vi "Wash Display Console View.vi"(8 "error in (no error)":errorcluster, 11 "View Model":T2) -> (0 "error out":errorcluster)   [LabVIEW 2017]
doc: "Contains set of indicators for demonstrate current state of Car Wash process."
uses:
  View Model/Controls/View Model.ctl
  Configuration Database/Controls/Config Model.ctl
  Configuration Database/Controls/Config Commands.ctl
  Configuration Database/Controls/Congif Data.ctl
  View Model/Controls/Shared Model.ctl
  Error Handler/Controls/Error Model.ctl
  Error Handler/Controls/Error Data.ctl
  Error Handler/Controls/Error Type.ctl
  Car Wash Controller/Controls/Car Wash Model.ctl
  Car Wash Controller/Controls/Controller Overhead.ctl
  Car Wash Controller/Controls/Vehicle Location.ctl
  Car Wash Controller/Controls/Car Wash States.ctl
  Car Wash Controller/Controls/CarWash CMD.ctl
  Controls/Car Wash Indicators.ctl
panel:
  out "Time Remaining":dbl format="%07.2g"
  out "Vehicle Out of Position":bool
  out "Wash Entry":bool
  out "Car Wash Indicators":T1
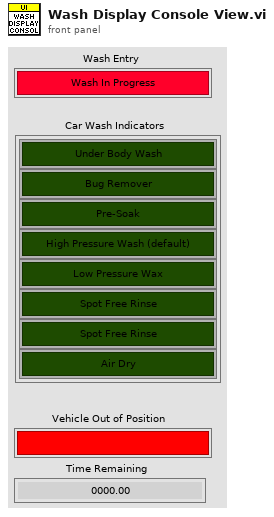
[diagram p1: front panel]
types:
  T1 = typedef "Car Wash Indicators.ctl" = cluster{"Under Body Wash":bool, "Bug Remover":bool, "Pre-Soak":bool, "High Pressure Wash":bool, "Low Pressure Wax":bool, "Spot Free Rinse":bool, "Tire Shine Foam":bool, "Air Dry":bool}
  T2 = typedef "View Model.ctl" = cluster{"Config Model":T3, "Shared Model":T4, "Error Model":T5, "Car Wash Model":T6}
  T3 = typedef "Config Model.ctl" = cluster{"Config CMD":refnum<user-event>, "Config Locked?":refnum<data-value>, "Config DVR":refnum<data-value>}
  T4 = typedef "Shared Model.ctl" = cluster{"Stop event":refnum<user-event>, "Stop DVR":refnum<data-value>}
  T5 = typedef "Error Model.ctl" = cluster{"Error event":refnum<user-event>}
  T6 = typedef "Car Wash Model.ctl" = cluster{"Out of Position Change":refnum<user-event>, "Wash Entry Change":refnum<user-event>, "Contr Overhead DVR":refnum<data-value>, "CarWash CMD":refnum<user-event>, "Location Change":refnum<user-event>, "Car Wash LEDs Change":refnum<user-event>}
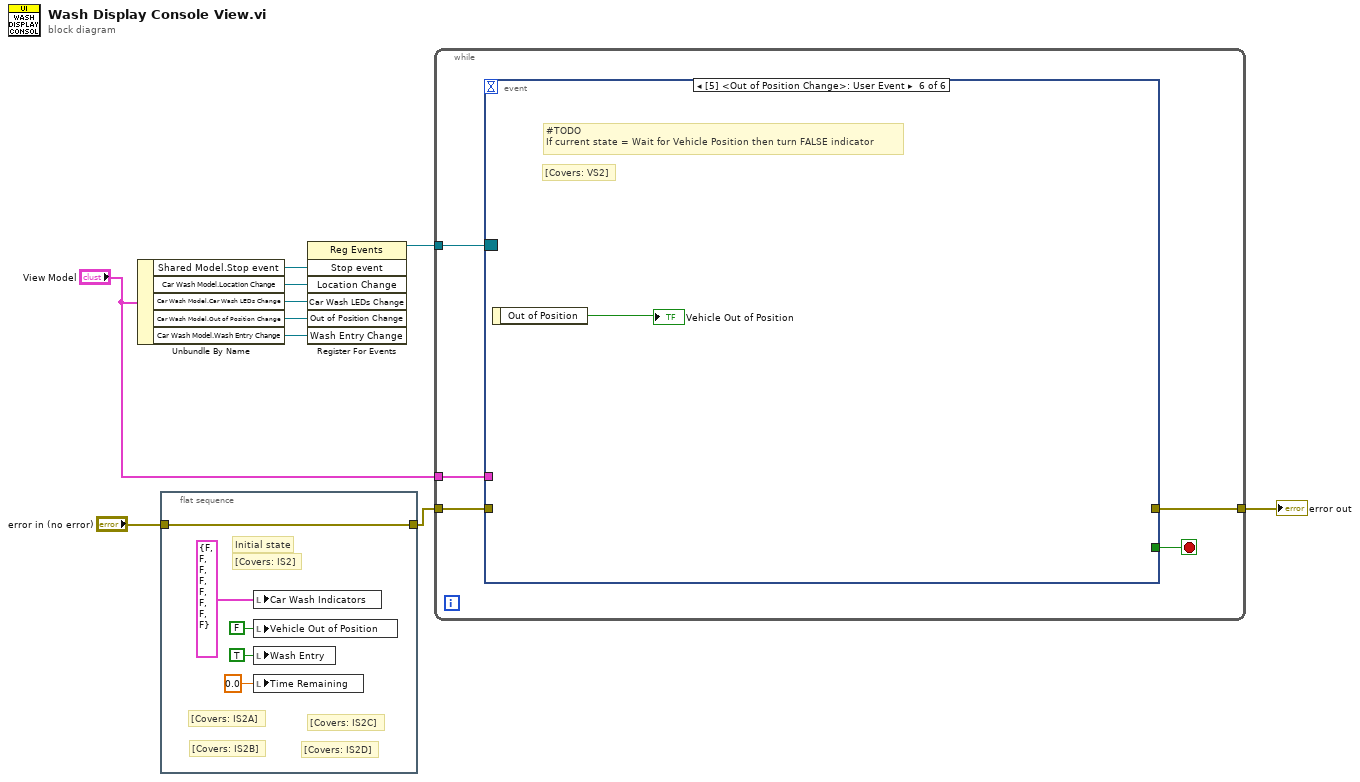
[diagram p0: block diagram]
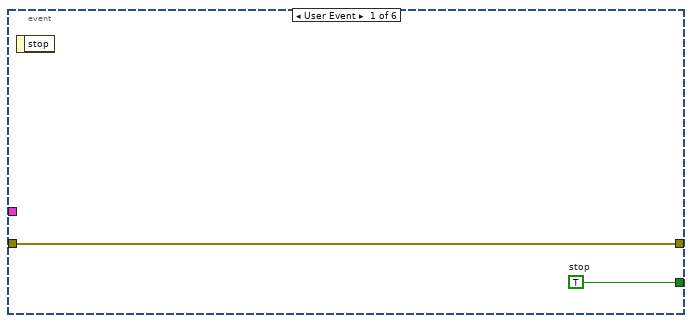
[diagram p2: hidden frame]
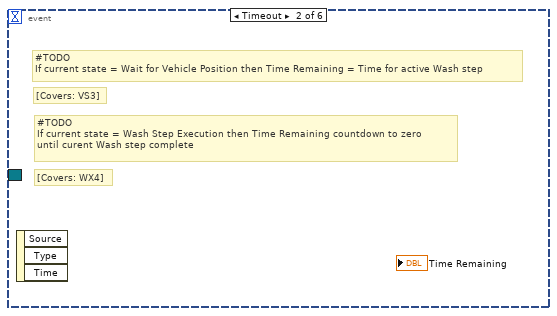
[diagram p3: hidden frame]
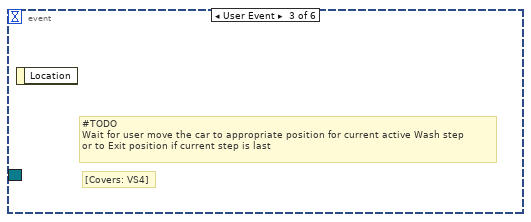
[diagram p4: hidden frame]
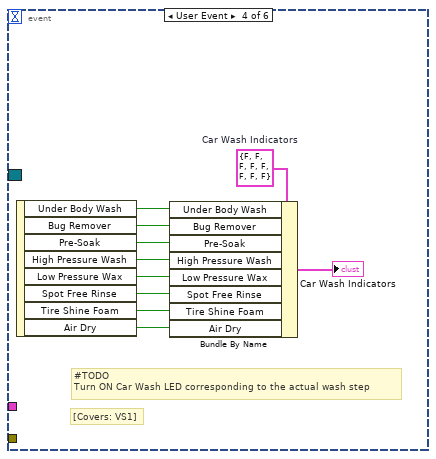
[diagram p5: hidden frame]
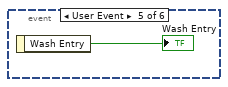
[diagram p6: hidden frame]
diagram:
  n1 = Unbundle By Name("View Model") -> ("Shared Model.Stop event"=w8:refnum<user-event>, "Car Wash Model.Location Change"=w7:refnum<user-event>, "Car Wash Model.Car Wash LEDs Change"=w3:refnum<user-event>, "Car Wash Model.Out of Position Change"=w2:refnum<user-event>, "Car Wash Model.Wash Entry Change"=w1:refnum<user-event>)
  n2 = flat-sequence {
    tunnel: "error in (no error)" -> [w11]
    tunnel: [w11] -> w4
    frame #0 {
      # "[Covers: IS2D]"
      # "[Covers: IS2C]"
      # "[Covers: IS2B]"
      # "[Covers: IS2A]"
      # "[Covers: IS2]"
      # "Initial state"
      n3 = local write "Car Wash Indicators"(T1 {"Under Body Wash"=FALSE, "Bug Remover"=FALSE, "Pre-Soak"=FALSE, "High Pressure Wash"=FALSE, "Low Pressure Wax"=FALSE, "Spot Free Rinse"=FALSE, "Tire Shine Foam"=FALSE, "Air Dry"=FALSE} ("Car Wash Indicators")) -> ()
      n4 = local write "Vehicle Out of Position"(FALSE ("Vehicle Out of Position")) -> ()
      n5 = local write "Wash Entry"(TRUE ("Wash Entry")) -> ()
      n6 = local write "Time Remaining"(0.0 ("Time Remaining")) -> ()
    }
  }
  n7 = register-events(w8, w7, w3, w2, w1) -> (reference out=w10:refnum<event-registration>)  [unwired: 2 in, 1 out]
  n8 = while {
    tunnel: w10 -> [w20]
    tunnel: w4 -> [w18]
    tunnel: [w17] -> w9
    tunnel: "View Model" -> [w16]
    stop <- w19 stop-if-true
    n9 = event shown="[5] <Out of Position Change>: User Event" {
      selector: w20 -> [_ _ _ _ _ _]
      dyn-events: _ -> [_ _ _ _ _ _]
      timeout: _ -> [_ _ _ _ _ _]
      tunnel: [w22 _ _ _ _ _] -> w19
      tunnel: w18 -> [w21 _ _ _ _ _]
      tunnel: [w21 _ _ _ _ _] -> w17
      tunnel: w16 -> [_ _ _ _ _ _]
      event User Event {
        w22 = TRUE  # stop
        n10 = event-data() -> ()  [unwired: 1 in, 1 out]
      }
      event Timeout {
        # "[Covers: WX4]"
        # "#TODO\nIf current state = Wash Step Execution then Time Remaining countdown to zero\nuntil curent Wash step complete"
        # "[Covers: VS3]"
        # "#TODO\nIf current state = Wait for Vehicle Position then Time Remaining = Time for active Wash step"
        n11 = event-data() -> ()  [unwired: 1 in, 3 out]
      }
      event User Event {
        # "[Covers: VS4]"
        # "#TODO\nWait for user move the car to appropriate position for current active Wash step\nor to Exit position if current step is last"
        n12 = event-data() -> ()  [unwired: 1 in, 1 out]
      }
      event User Event {
        w24 = T1 {"Under Body Wash"=FALSE, "Bug Remover"=FALSE, "Pre-Soak"=FALSE, "High Pressure Wash"=FALSE, "Low Pressure Wax"=FALSE, "Spot Free Rinse"=FALSE, "Tire Shine Foam"=FALSE, "Air Dry"=FALSE}  # Car Wash Indicators
        # "[Covers: VS1]"
        # "#TODO\nTurn ON Car Wash LED corresponding to the actual wash step"
        n13 = event-data() -> ("Under Body Wash"=w32:bool, "Bug Remover"=w31:bool, "Pre-Soak"=w30:bool, "High Pressure Wash"=w29:bool, "Low Pressure Wax"=w28:bool, "Spot Free Rinse"=w27:bool, "Tire Shine Foam"=w26:bool, "Air Dry"=w25:bool)  [unwired: 1 in]
        n14 = Bundle By Name(cluster=w24, "Under Body Wash"=w32, "Bug Remover"=w31, "Pre-Soak"=w30, "High Pressure Wash"=w29, "Low Pressure Wax"=w28, "Spot Free Rinse"=w27, "Tire Shine Foam"=w26, "Air Dry"=w25) -> (→"Car Wash Indicators":T1)
      }
      event User Event {
        n15 = event-data() -> ("Wash Entry"=→"Wash Entry":bool)  [unwired: 1 in]
      }
      event User Event {
        # "[Covers: VS2]"
        # "#TODO\nIf current state = Wait for Vehicle Position then turn FALSE indicator"
        n16 = event-data() -> ("Out of Position"=→"Vehicle Out of Position":bool)  [unwired: 1 in]
      }
    }
  }
  "error out" <- w9
